vi "Wait_NoBytes.vi"(8 "error in (no error)":errorcluster, 10 "milliseconds to wait":u32=100, 11 "Server":path) -> (0 "error out":errorcluster, 3 "String":string)   [LabVIEW 2020]
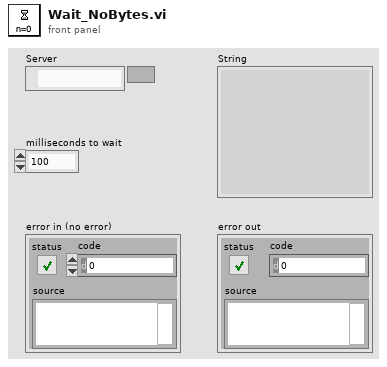
[diagram p1: front panel]
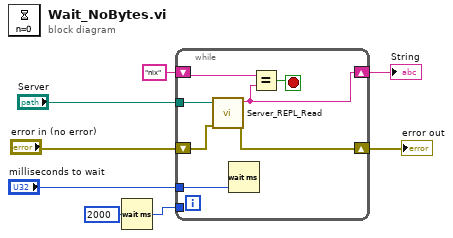
[diagram p0: block diagram]
diagram:
  n1 = Wait (ms)(milliseconds to wait=u32 2000) -> (millisecond timer value=w3:u32)
  n2 = while {
    tunnel: "Server" -> [w13]
    shift-right: [w14] -> w7
    shift-left: "error in (no error)" -> [w15]
    shift-right: [w10] -> w6
    shift-left: "nix" -> [w11]
    tunnel: w3 -> [_]
    tunnel: "milliseconds to wait" -> [w9]
    stop <- w12 stop-if-true
    n3 = call "Server_REPL_Read.vi"("error in (no error)"=w15, "Server"=w13) -> ("error out"=w14:errorcluster, "REPL"=w10:string)  [unwired: 7 in, 1 out]
    n4 = Wait (ms)(milliseconds to wait=w9) -> ()  [unwired: 1 out]
    n5 = Equal?(x=w11, y=w10) -> (x = y?=w12:bool)
  }
  "error out" <- w7
  "String" <- w6
